vi "Recursive file list.vi"(8 "error in (no error)":errorcluster, 10 "Path":string, 11 "FTP in":refnum<class "FTP.lvclass">) -> (0 "error out":errorcluster, 1 "Files":string[](array[string]), 2 "Directories":string[](array[string]), 3 "FTP out":refnum<class "FTP.lvclass">)   [LabVIEW 2015, in "RT Management.lvlib" / "FTP.lvclass"]
uses:
  FTP.lvclass
  FTP.lvclass/FTP.ctl
  Get Session.vi
  <vilib>/Utility/error.llb/Trim Whitespace.vi
  File Transfer Behavior/File Transfer Behavior.lvclass
  <vilib>/FTP/NI_FTP.lvlib
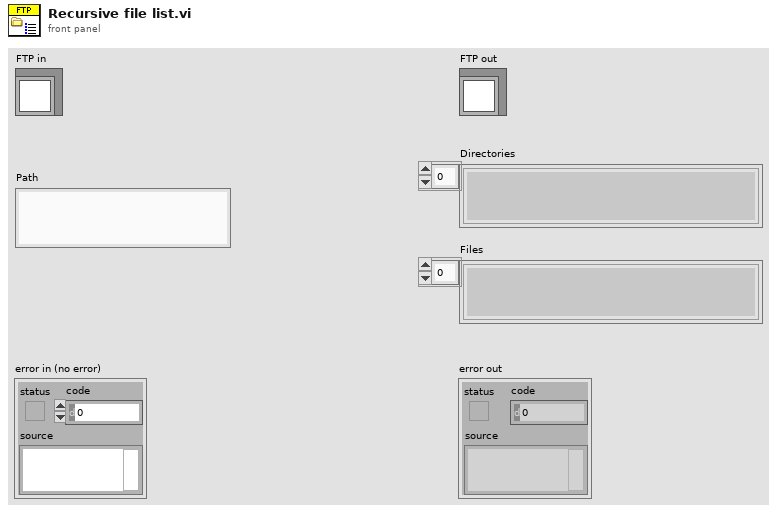
[diagram p1: front panel]
types:
  T1 = typedef "NI_FTP.lvlib/FTP Session.ctl" = refnum<k5>
  T2 = typedef "NI_FTP.lvlib/FTP File Info.ctl" = cluster{"type":enum16{"unknown", "file", "dir", "link"}, "permissions":string, "owner":string, "group":string, "size":i32, "date":string, "name":string, "link name":string}
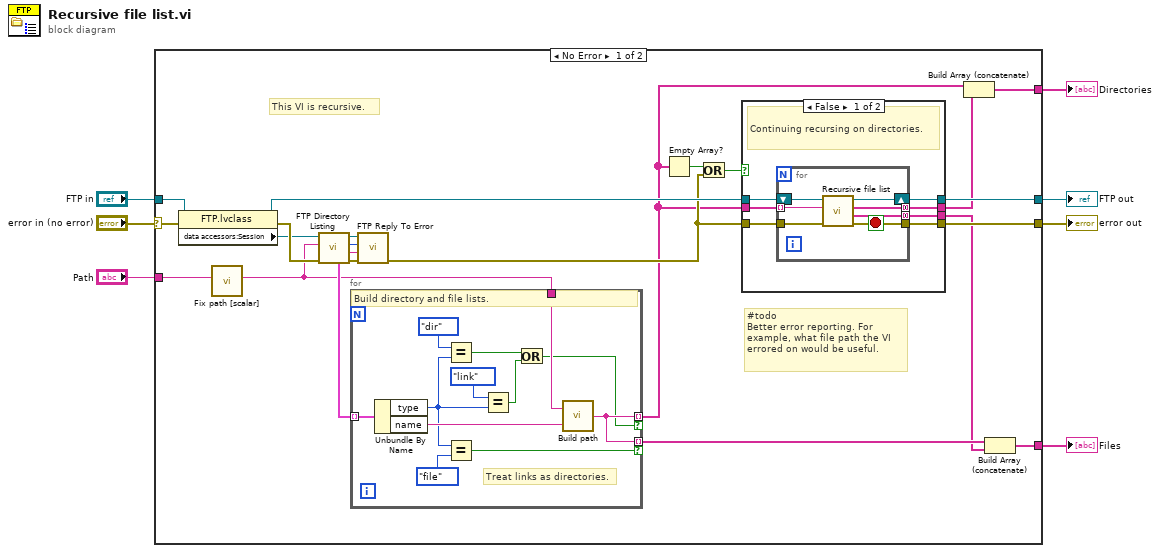
[diagram p0: block diagram]
diagram:
  n1 = case shown="No Error" "error in (no error)" {
    selector: "error in (no error)" -> [w14 w60]
    tunnel: [w29 w60] -> w6
    tunnel: [w20 w59] -> w4
    tunnel: "FTP in" -> [w28 w59]
    tunnel: "Path" -> [w9 _]
    tunnel: [w17 _] -> w2
    tunnel: [w15 _] -> w1
    frame No Error {
      # "This VI is recursive."
      # "#todo\nBetter error reporting. For example, what file path the VI errored on would be useful."
      n2 = property class="FTP.lvclass"(reference=w28, error in=w14) -> (reference out=w21:refnum<class "FTP.lvclass">, error out=w30:errorcluster, "data accessors:Session"=w27:T1)
      n3 = call "Fix path [scalar].vi"("Path in"=w9) -> ("Path out"=w8:string)  [unwired: 8 in, 2 out]
      n4 = call <vilib>:"FTP Directory Listing.vi"("error in (no error)"=w30, "directory path"=w8, "ftp session"=w27) -> ("error out"=w26:errorcluster, "reply string"=w25:string, "reply code"=w24:i32, "ftp session out"=w23:T1, "dir list"=w22:T2[])  [unwired: 4 in]
      n5 = for {
        tunnel: w22 -> [w57] mode=indexing
        tunnel: w8 -> [w55]
        tunnel: [w54] -> w10 mode=indexing if=w47
        tunnel: [w54] -> w19 mode=indexing if=w53
        # "Treat links as directories."
        # "Build directory and file lists."
        n6 = Unbundle By Name(w57) -> ("type"=w51:enum16{"unknown", "file", "dir", "link"}, "name"=w56:string)
        n7 = Equal?(x=enum16{"unknown", "file", "dir", "link"}."dir" ("type"), y=w51) -> (x = y?=w49:bool)
        n8 = Equal?(x=w51, y=enum16{"unknown", "file", "dir", "link"}."file" ("type")) -> (x = y?=w53:bool)
        n9 = Equal?(x=enum16{"unknown", "file", "dir", "link"}."link" ("type"), y=w51) -> (x = y?=w48:bool)
        n10 = Or(x=w49, y=w48) -> (x .or. y?=w47:bool)
        n11 = call "Build path.vi"("Relative path"=w56, "Base path"=w55) -> ("Resulting path"=w54:string)
      }
      n12 = call <vilib>:"FTP Reply To Error.vi"("error in (no error)"=w26, "reply string in"=w25, "reply code in"=w24, "ftp session"=w23) -> ("error out"=w12:errorcluster)  [unwired: 3 out]
      n13 = Empty Array?(array=w10) -> (empty?=w13:bool)
      n14 = Or(x=w13, y=w12) -> (x .or. y?=w11:bool)
      n15 = case shown="False" w11 {
        tunnel: [w31 w45] -> w29
        tunnel: w12 -> [w37 w45]
        tunnel: w21 -> [w36 w46]
        tunnel: [w35 w46] -> w20
        tunnel: [w34 _] -> w18
        tunnel: [w33 _] -> w16
        tunnel: w10 -> [w32 _]
        frame False {
          # "Continuing recursing on directories."
          n16 = for {
            tunnel: [w41] -> w34 mode=concatenating
            tunnel: [w40] -> w33 mode=concatenating
            tunnel: w32 -> [w39] mode=indexing
            tunnel: w37 -> [w44]
            tunnel: [w38] -> w31
            shift-right: [w42] -> w35
            shift-left: w36 -> [w43]
            stop <- w38 stop-if-true
            n17 = call-dynamic "Recursive file list.vi"("error in (no error)"=w44, "Path"=w39, "FTP in"=w43) -> ("error out"=w38:errorcluster, "Files"=w41:string[], "Directories"=w40:string[], "FTP out"=w42:refnum<class "FTP.lvclass">)  [unwired: 5 in]
          }
        }
        frame True {
          # "Directory array is empty or an error occurred. Stop recursion."
        }
      }
      n18 = Build Array (concatenate)(w10, w16) -> (w15:string[])
      n19 = Build Array (concatenate)(w19, w18) -> (w17:string[])
    }
    frame Error {
    }
  }
  "error out" <- w6
  "FTP out" <- w4
  "Files" <- w2
  "Directories" <- w1
